vi "niRFSTS Sequence Flow Insert Measurements.vi"(0 "Session Handle in":T1, 5 "Measurement Insertion Progress":refnum<vi>, 11 "error in (no error)":errorcluster) -> (4 "Session Handle out":T1, 15 "error out":errorcluster)   [LabVIEW 2018, in "niRFSTS Sequence Flow.lvclass"]
uses:
  niRFSTS Sequence Flow.lvclass
  Typedefs/Session Handle.ctl
  niRFSTS Sequence Flow.lvclass/niRFSTS Sequence Flow.ctl
  Plugins/Measurement Interface.lvlibp/Public Methods/Sequence Reference/Write Sequence Reference.vi
  Plugins/Measurement Interface.lvlibp/Private Methods/Measurement Name/Write Measurement Name.vi
  Plugins/Measurement Interface.lvlibp/Measurement Interface.lvclass
  Plugins/TestStand API Tools (TSAT).lvlibp/TSAT Examples/TSAT Examples.lvlib
  Plugins/TestStand API Tools (TSAT).lvlibp/Sequence Actions/TSAT Sequence Actions.lvlib
  Plugins/TestStand API Tools (TSAT).lvlibp/Step Actions/TSAT Step Actions.lvlib
  Plugins/Measurement Data.lvlibp/Measurement Data.lvclass
  Plugins/TestStand API Tools (TSAT).lvlibp/Sequence File Actions/TSAT Sequence File Actions.lvlib
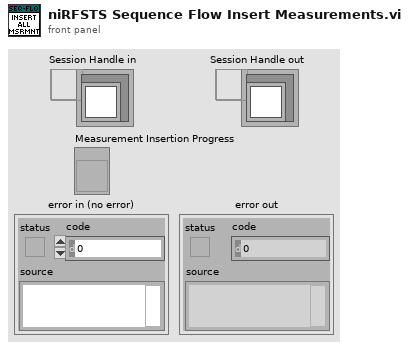
[diagram p1: front panel]
types:
  T1 = typedef "niRFSTS Sequence Flow.lvclass/Session Handle.ctl" = refnum<data-value>
  T2 = typedef "File Parsing Interface.lvlibp/File Parsing Interface.lvclass/Parsed Measurement.ctl" = cluster{"Test Mode":string, "Measurement Data Out":refnum<class "Measurement Data.lvclass">}
  T3 = typedef "Measurement Data.lvlibp/Measurement Data.lvclass/Measurement Description.ctl" = cluster{"Measurement Sequence Position":T4, "Measurement Data":refnum<class "String Database.lvclass">, "Measurement Definition Entry":string}
  T4 = typedef "Measurement Data.lvlibp/Measurement Data.lvclass/Measurement Position.ctl" = enum16{"PreMeasurement", "MainMeasurement", "PostMeasurement"}
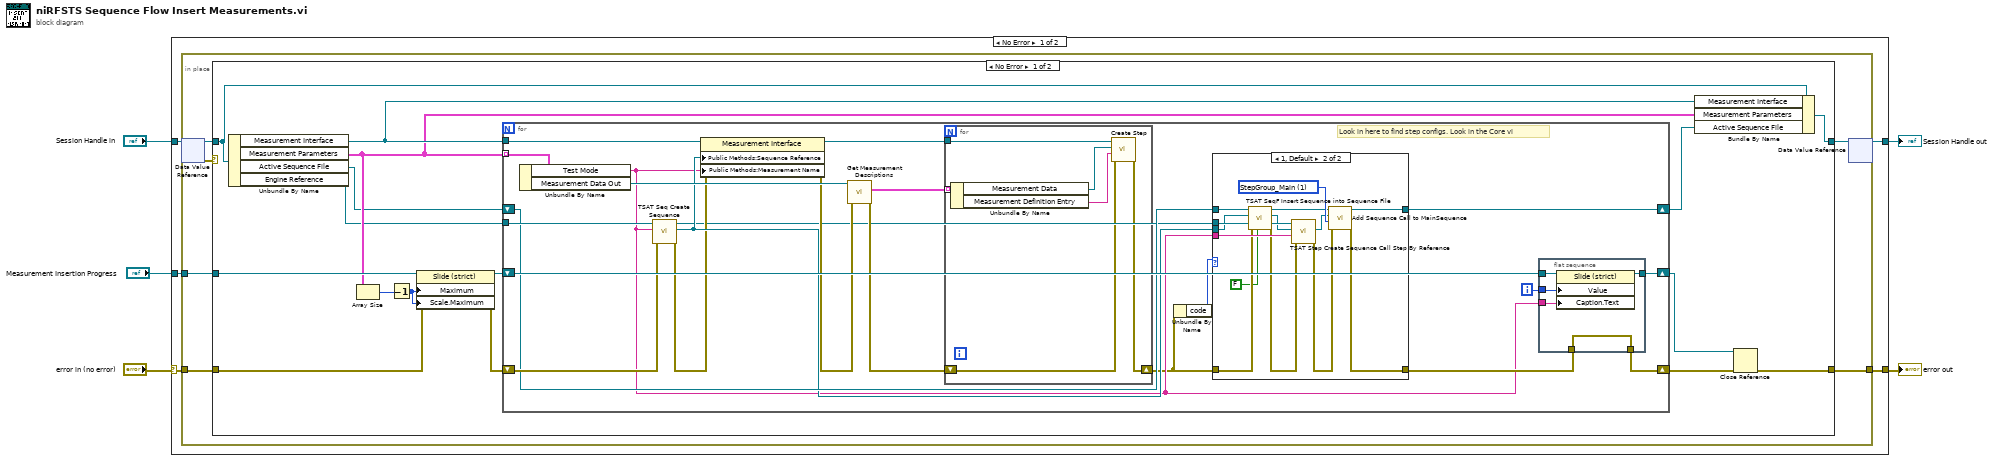
[diagram p0: block diagram]
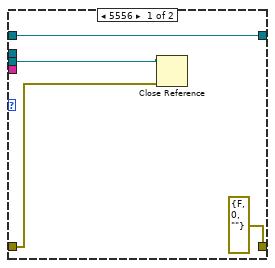
[diagram p2: hidden frame]
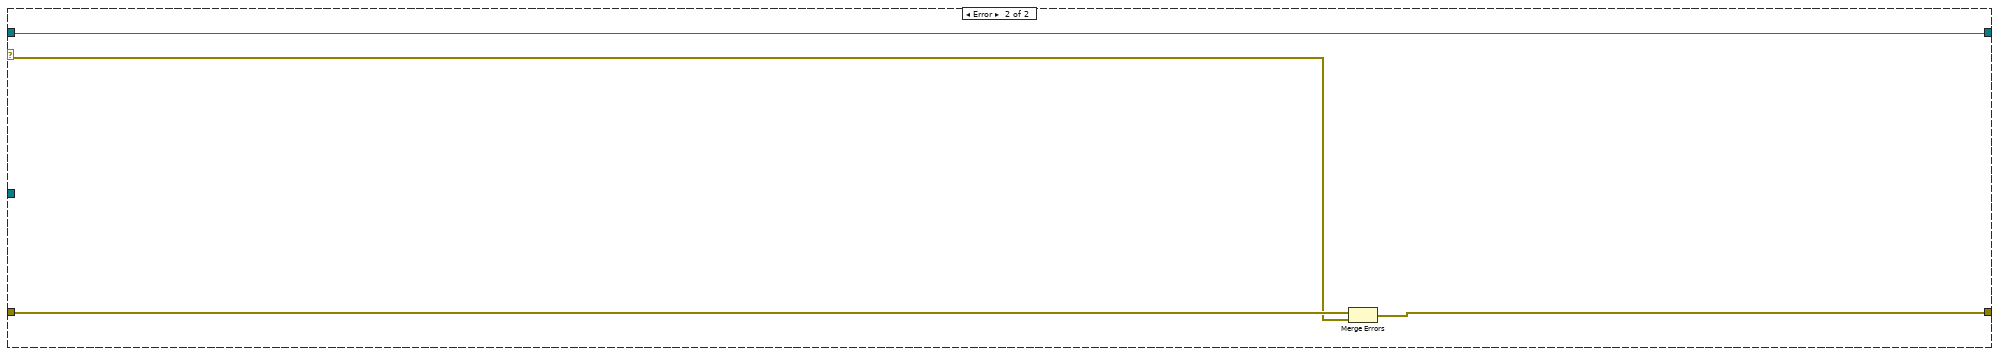
[diagram p3: hidden frame]
diagram:
  n1 = case shown="No Error" "error in (no error)" {
    selector: "error in (no error)" -> [w8 w88]
    tunnel: "Session Handle in" -> [w10 w89]
    tunnel: [w9 w89] -> w4
    tunnel: [w7 w88] -> w3
    tunnel: "Measurement Insertion Progress" -> [w6 _]
    frame No Error {
      n2 = in-place {
        in-place-border: w8 -> [w12]
        in-place-border: [w15] -> w7
        in-place-border: w6 -> [w11]
        n3 = in-place-dvr #1(w10) -> (w16:refnum<class "niRFSTS Sequence Flow.lvclass">, w13:errorcluster)
        n4 = case shown="No Error" w13 {
          selector: w13 -> [_ w86]
          tunnel: w16 -> [w32 w84]
          tunnel: [w23 w85] -> w15
          tunnel: [w31 w84] -> w14
          tunnel: w12 -> [w27 w87]
          tunnel: w11 -> [w28 _]
          frame No Error {
            n5 = Unbundle By Name(w32) -> ("Measurement Interface"=w29:refnum<class "Measurement Interface.lvclass">, "Measurement Parameters"=w25:T2[], "Active Sequence File"=w18:refnum<k7>, "Engine Reference"=w17:refnum<k7>)
            n6 = Array Size(array=w25) -> (size(s)=w21:i32)
            n7 = Decrement(x=w21) -> (x-1=w20:i32)
            n8 = property class="Slide (strict)"(reference=w28, error in=w27, "Maximum"=w20, "Scale.Maximum"=w20) -> (reference out=w24:refnum<vi>, error out=w26:errorcluster)
            n9 = for {
              shift-right: [w53] -> w30
              shift-left: w26 -> [w44]
              shift-right: [w54] -> w19
              shift-left: w18 -> [w39]
              tunnel: w25 -> [w46] mode=indexing
              tunnel: w29 -> [w48]
              shift-right: [w51] -> w22
              shift-left: w24 -> [w52]
              tunnel: w17 -> [w45]
              i -> [w50]
              # "Look in here to find step configs. Look in the Core vi"
              n10 = Unbundle By Name(w46) -> ("Test Mode"=w35:string, "Measurement Data Out"=w43:refnum<class "Measurement Data.lvclass">)
              n11 = call "TSAT Seq Create Sequence.vi"("Error in"=w44, "Sequence Name"=w35, "Engine In"=w45) -> ("Error out"=w37:errorcluster, "Sequence Reference Out"=w38:refnum<k7>, "Engine Out"=w36:refnum<k7>)  [unwired: 6 in]
              n12 = property class="Measurement Interface"(reference=w48, error in=w37, "Public Methods:Sequence Reference"=w38, "Public Methods:Measurement Name"=w35) -> (reference out=w47:refnum<class "Measurement Interface.lvclass">, error out=w42:errorcluster)
              n13 = call "Get Measurement Descriptions.vi"("error in (no error)"=w42, "Measurement Data in"=w43) -> ("error out"=w41:errorcluster, "Measurement Step Descriptions"=w40:T3[])  [unwired: 7 in, 1 out]
              n14 = for {
                tunnel: w47 -> [w77]
                shift-right: [w78] -> w34
                shift-left: w41 -> [w75]
                tunnel: w40 -> [w76] mode=indexing
                n15 = Unbundle By Name(w76) -> ("Measurement Data"=w74:refnum<class "String Database.lvclass">, "Measurement Definition Entry"=w73:string)
                n16 = call-dynamic "Create Step.vi"("error in (no error)"=w75, "Measurement Definition Entry"=w73, "Measurement Parameters In"=w74, "Measurement Interface in"=w77) -> ("error out"=w78:errorcluster)  [unwired: 6 in, 1 out]
              }
              n17 = Unbundle By Name(w34) -> ("code"=w33:i32)
              n18 = case shown="1, Default" w33 {
                tunnel: [w58 w72] -> w54
                tunnel: [errorcluster {"status"=FALSE, "code"=0, "source"=""} ("Error Out") w70] -> w49
                tunnel: w39 -> [w58 w60]
                tunnel: w38 -> [w57 w62]
                tunnel: w36 -> [_ w67]
                tunnel: w35 -> [_ w66]
                tunnel: w34 -> [w56 w65]
                frame 5556 {
                  n19 = Close Reference(reference=w57, error in (no error)=w56) -> ()  [unwired: 1 out]
                }
                frame 1, Default {
                  w71 = 1 items=["StepGroup_Setup", "StepGroup_Main", "StepGroup_Cleanup"] ("Step Group")
                  n20 = call "TSAT SeqF Insert Sequence into Sequence File.vi"("Close Sequence Reference?(T)"=FALSE, "Error in"=w65, "Sequence to Insert"=w62, "Sequence File"=w60) -> ("Error Out"=w64:errorcluster, "Sequence Reference Out"=w61:refnum<k7>, "Sequence File Out"=w59:refnum<k7>)  [unwired: 5 in]
                  n21 = call "TSAT Step Create Sequence Call Step By Reference.vi"("Error In"=w64, "Step Name"=w66, "Sequence to Call"=w61, "Engine In"=w67) -> ("Error Out"=w69:errorcluster, "Step Reference"=w68:refnum<k7>)  [unwired: 5 in, 1 out]
                  n22 = call "Add Sequence Call to MainSequence.vi"("Error In"=w69, "Step Group"=w71, "Step In"=w68, "Sequence File In"=w59) -> ("Error Out"=w70:errorcluster, "Sequence File Out"=w72:refnum<k7>)  [unwired: 6 in]
                }
              }
              n23 = flat-sequence {
                tunnel: w52 -> [w83]
                tunnel: [w81] -> w53
                tunnel: [w82] -> w51
                tunnel: w50 -> [w80]
                tunnel: w49 -> [w81]
                tunnel: w35 -> [w79]
                frame #0 {
                  n24 = property class="Slide (strict)"(reference=w83, "Value"=w80, "Caption.Text"=w79) -> (reference out=w82:refnum<vi>)  [unwired: 1 in, 1 out]
                }
              }
            }
            n25 = Bundle By Name(cluster=w32, "Measurement Interface"=w29, "Measurement Parameters"=w25, "Active Sequence File"=w19) -> (w31:refnum<class "niRFSTS Sequence Flow.lvclass">)
            n26 = Close Reference(reference=w22, error in (no error)=w30) -> (error out=w23:errorcluster)
          }
          frame Error {
            n27 = Merge Errors(w87, w86) -> (w85:errorcluster)
          }
        }
        n28 = in-place-dvr #1(w14) -> (w9:T1)  [unwired: 1 out]
      }
    }
    frame Error {
    }
  }
  "Session Handle out" <- w4
  "error out" <- w3
